vi "Ethernet Reader.vi"(0 "IP":string, 1 "포트":u16=50, 3 "에러 입력(에러 없음)":errorcluster) -> (4 "Axis":string, 6 "L":i32, 7 "R":i32, 8 "C":i32, 9 "에러 출력":errorcluster)   [LabVIEW 2013]
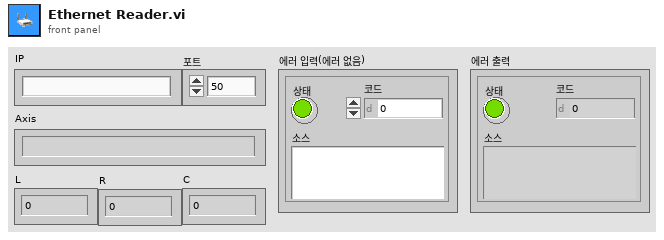
[diagram p1: front panel]
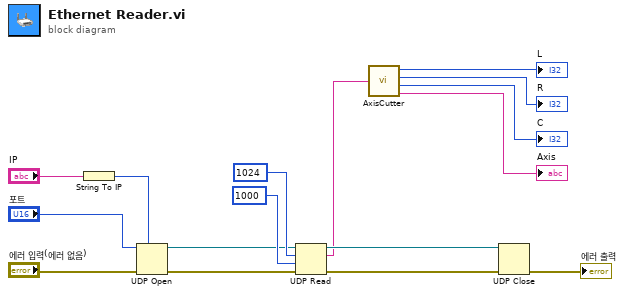
[diagram p0: block diagram]
diagram:
  n1 = String To IP(1:"IP") -> (0:w10:u32)
  n2 = UDP Open(7:w10, 8:"에러 입력(에러 없음)", 11:"포트") -> (port=w6:refnum<k16>, 0:w7:errorcluster)  [unwired: 2 in, 1 out]
  n3 = UDP Read(connection ID=w6, max size (548)=1024 ("최대 크기(548)"), timeout ms (25000)=1000 ("타임아웃 ms (25000)"), 8:w7) -> (data out=w5:string, error out=w14:errorcluster, 3:w13:refnum<k16>)  [unwired: 2 out]
  n4 = call "AxisCutter.vi"("수신"=w5) -> ("L"=→"L":i32, "R"=→"R":i32, "C"=→"C":i32, "Axis"=→"Axis":string)
  n5 = UDP Close(connection ID=w13, 8:w14) -> (error out=→"에러 출력":errorcluster)  [unwired: 1 out]
